vi "Strip Duplicate Events.vi"(11 "Array in":string[][](array[string])) -> (1 "Duplicates Removed":i16, 2 "Remaining \"3-Events\"":i32, 3 "Array out":string[][](array[string]))   [LabVIEW 2019, in "Muon Data Post-Processing.lvlib"]
uses:
  Muon Data Post-Processing.lvlib
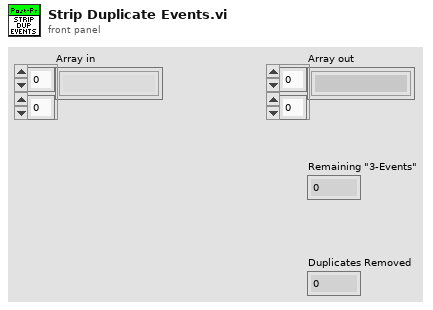
[diagram p1: front panel]
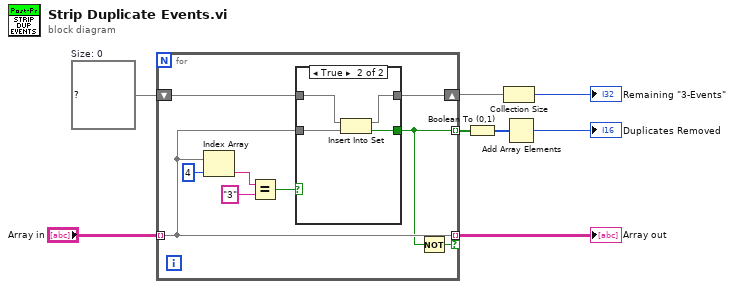
[diagram p0: block diagram]
diagram:
  w6 = set{string[]} {}  # Size: 0
  n1 = for {
    tunnel: "Array in" -> [w11] mode=indexing
    shift-right: [w12] -> w5
    shift-left: w6 -> [w13]
    tunnel: [w11] -> w8 mode=indexing if=w10
    tunnel: [w9] -> w2 mode=indexing
    n2 = Index Array(array=w11, index=4) -> (element=w16:string)
    n3 = Equal?(x=w16, y="3") -> (x = y?=w14:bool)
    n4 = case shown="True" w14 {
      tunnel: w11 -> [_ w22]
      tunnel: w13 -> [w18 w21]
      tunnel: [w18 w20] -> w12
      tunnel: [_ w19] -> w9
      frame False {
      }
      frame True {
        n5 = Insert Into Set(10:w22, 11:w21) -> (2:w19:bool, 3:w20:set{string[]})
      }
    }
    n6 = Not(x=w9) -> (.not. x?=w10:bool)
  }
  "Array out" <- w8
  n7 = Boolean To (0,1)(Boolean=w2) -> (0, 1=w3:i16[])
  n8 = Collection Size(1:w5) -> (0:→"Remaining \"3-Events\"":i32)
  n9 = Add Array Elements(numeric array=w3) -> (sum=→"Duplicates Removed":i16)
